vi "FPGA_buttonToLED.vi"   [LabVIEW 2018]
uses:
  <vilib>/rvi/Emulation/niFpgaGetClockAttributes.vi
  <vilib>/rvi/Emulation/niFpgaSctlEmulationGetInTimedLoop.vi
  <vilib>/rvi/Emulation/niFpgaEmulationReportErrorSimple.vi
  <vilib>/rvi/eio/common/nirviEmuTemplateMethod_errors.vi
  <vilib>/rvi/Emulation/niFpgaCriticalErrorInLSC.vi
  <vilib>/eio/EIONode/EIONode.xnode
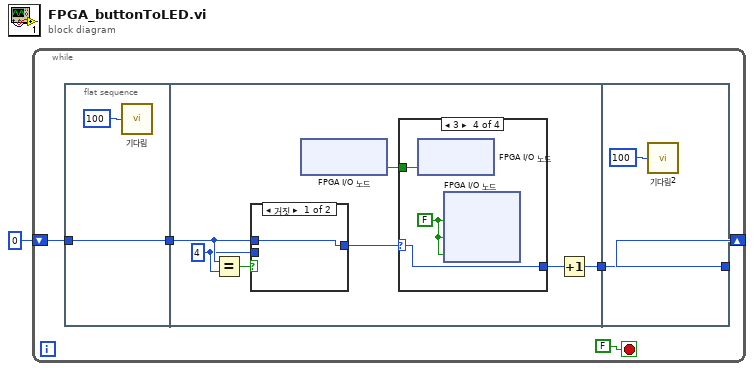
[diagram p0: block diagram]
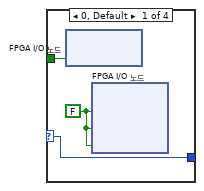
[diagram p2: hidden frame]
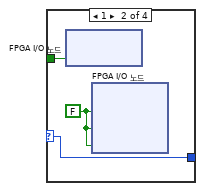
[diagram p3: hidden frame]
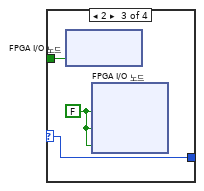
[diagram p4: hidden frame]
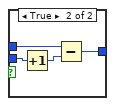
[diagram p5: hidden frame]
diagram:
  n1 = while {
    shift-right: [w5] -> _
    shift-left: i8 0 -> [w4]
    stop <- FALSE stop-if-true
    n2 = flat-sequence {
      tunnel: w4 -> [w8]
      tunnel: [w8] -> w3
      tunnel: w3 -> [w13]
      tunnel: [w15] -> w2
      tunnel: [w34] -> w5
      tunnel: w2 -> [w34]
      frame #0 {
        n3 = call "기다림"("Count(mSec)"=i8 100) -> ()  [unwired: 1 out]
      }
      frame #1 {
        w9 = i8 4 ("y")
        n4 = Equal?(x=w13, y=w9) -> (x = y?=w14:bool)
        n5 = case shown="거짓" w14 {
          tunnel: w13 -> [w28 w32]
          tunnel: w9 -> [_ w30]
          tunnel: [w28 w31] -> w11
          frame False {
          }
          frame True {
            n6 = Increment(x=w30) -> (x+1=w29:i8)
            n7 = Subtract(x=w32, y=w29) -> (x-y=w31:i8)
          }
        }
        n8 = xnode "FPGA I/O 노드"() -> ("Button0"=w12:bool)  [unwired: 1 in, 1 out]
        n9 = case shown="3" w11 {
          selector: w11 -> [w17 w20 w23 w26]
          tunnel: w12 -> [w18 w21 w24 w27]
          tunnel: [w17 w20 w23 w26] -> w10
          frame 0, Default {
            w16 = FALSE
            n10 = xnode "FPGA I/O 노드"("LED0"=w18) -> ()  [unwired: 1 in, 1 out]
            n11 = xnode "FPGA I/O 노드"("LED3"=w16, "LED1"=w16, "LED2"=w16) -> ()  [unwired: 3 in, 3 out]
          }
          frame 1 {
            w19 = FALSE
            n12 = xnode "FPGA I/O 노드"("LED1"=w21) -> ()  [unwired: 1 in, 1 out]
            n13 = xnode "FPGA I/O 노드"("LED3"=w19, "LED0"=w19, "LED2"=w19) -> ()  [unwired: 3 in, 3 out]
          }
          frame 2 {
            w22 = FALSE
            n14 = xnode "FPGA I/O 노드"("LED2"=w24) -> ()  [unwired: 1 in, 1 out]
            n15 = xnode "FPGA I/O 노드"("LED3"=w22, "LED1"=w22, "LED0"=w22) -> ()  [unwired: 3 in, 3 out]
          }
          frame 3 {
            w25 = FALSE
            n16 = xnode "FPGA I/O 노드"("LED3"=w27) -> ()  [unwired: 1 in, 1 out]
            n17 = xnode "FPGA I/O 노드"("LED0"=w25, "LED1"=w25, "LED2"=w25) -> ()  [unwired: 3 in, 3 out]
          }
        }
        n18 = Increment(x=w10) -> (x+1=w15:i8)
      }
      frame #2 {
        n19 = call "기다림2"("Count(mSec)"=i8 100) -> ()  [unwired: 1 out]
      }
    }
  }
